vi "_TreeItem.Property.Set.Dictionary.Info.vi"(8 "error in":errorcluster, 11 "Variant":variant) -> (0 "error out":errorcluster, 1 "Dictionary?":bool, 2 "Dictionary Info":T1, 3 "Variant out":variant)   [LabVIEW 2027, in "Advanced System Definition.lvlib"]
uses:
  <vilib>/NI/NI VeriStand Advanced SysDef API/SysDef API/Advanced System Definition.lvlib
  _Types/Property.Dictionary.ctl
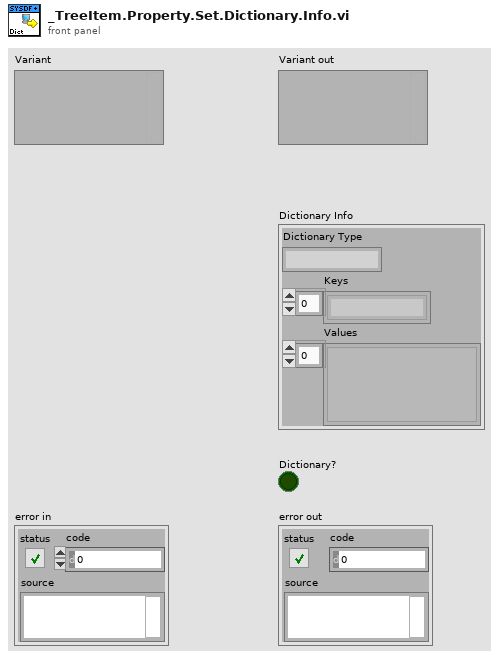
[diagram p1: front panel]
types:
  T1 = typedef "Advanced System Definition.lvlib/Property.Dictionary.ctl" = cluster{"Dictionary Type":string, "Keys":string[], "Values":variant[]}
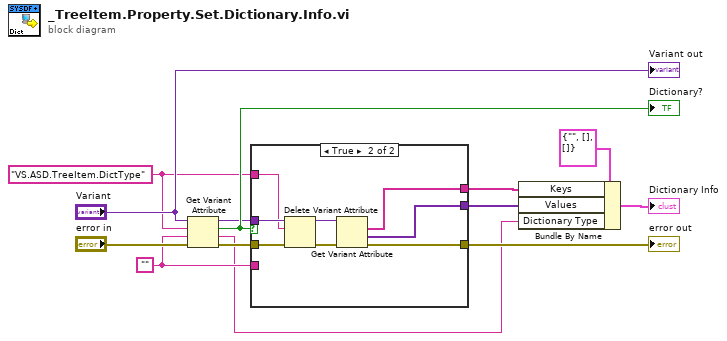
[diagram p0: block diagram]
diagram:
  w8 = ""
  w7 = "VS.ASD.TreeItem.DictType" ("name")
  n1 = Get Variant Attribute(Variant="Variant", name=w7, default value (empty Variant)=w8, error in="error in") -> (duplicate Variant=w9:variant, found=w11:bool, value=w4:string, error out=w10:errorcluster)
  "Dictionary?" <- w11
  n2 = case shown="True" w11 {
    tunnel: w10 -> [w14 w22]
    tunnel: w9 -> [_ w21]
    tunnel: w8 -> [_ _]
    tunnel: w7 -> [_ w20]
    tunnel: [_ w17] -> w3
    tunnel: [_ w16] -> w2
    tunnel: [w14 w15] -> w6
    frame False {
    }
    frame True {
      n3 = Delete Variant Attribute(4:w22, 6:w20, 7:w21) -> (0:w19:errorcluster, 3:w18:variant)  [unwired: 1 out]
      n4 = Get Variant Attribute(Variant=w18, error in=w19) -> (names=w17:string[], values=w16:variant[], error out=w15:errorcluster)  [unwired: 2 in, 1 out]
    }
  }
  "error out" <- w6
  n5 = Bundle By Name(cluster=T1 {"Dictionary Type"="", "Keys"=[], "Values"=[]} ("Dictionary"), "Keys"=w3, "Values"=w2, "Dictionary Type"=w4) -> (→"Dictionary Info":T1)
  "Variant out" <- "Variant"
